vi "GetStringFromRing.vi"(7 "Index":bool, 8 "error in (no error)":errorcluster, 10 "Select Asset":i32, 11 "Ring in":refnum<vi>) -> (0 "error out":errorcluster, 3 "String":string)   [LabVIEW 2019]
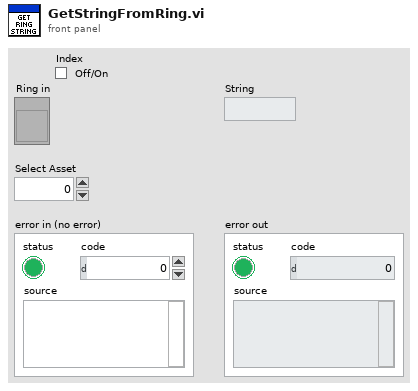
[diagram p1: front panel]
types:
  T1 = typedef "LVStringsAndValuesArrayTypeDef.ctl" = cluster{"String":string, "Value":ext}[]
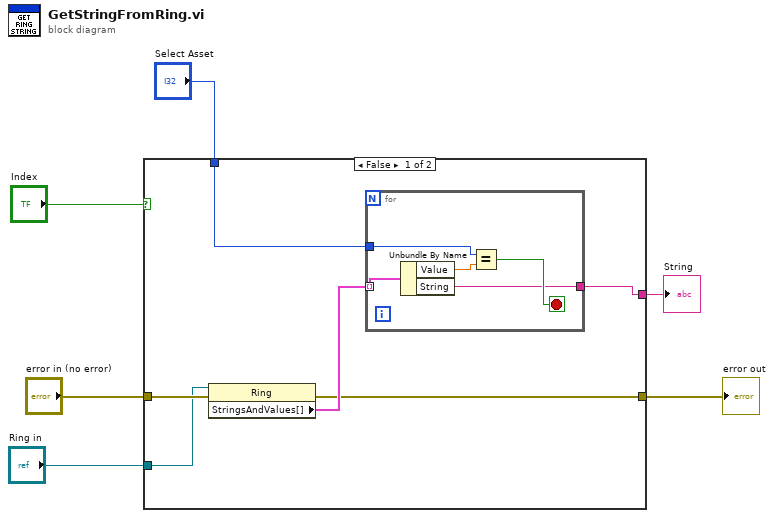
[diagram p0: block diagram]
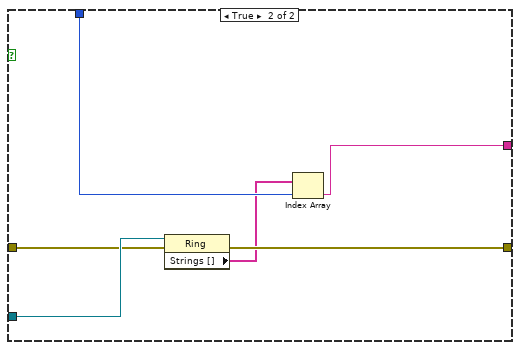
[diagram p2: hidden frame]
diagram:
  n1 = case shown="False" "Index" {
    tunnel: [w7 w23] -> w6
    tunnel: [w8 w22] -> w5
    tunnel: "Select Asset" -> [w9 w21]
    tunnel: "Ring in" -> [w11 w19]
    tunnel: "error in (no error)" -> [w12 w18]
    frame False {
      n2 = property class="Ring"(reference=w11, error in=w12) -> (error out=w7:errorcluster, "StringsAndValues[]"=w10:T1)  [unwired: 1 out]
      n3 = for {
        tunnel: w10 -> [w17] mode=indexing
        tunnel: w9 -> [w16]
        tunnel: [w13] -> w8
        stop <- w14 stop-if-true
        n4 = Unbundle By Name(w17) -> ("Value"=w15:ext, "String"=w13:string)
        n5 = Equal?(x=w16, y=w15) -> (x = y?=w14:bool)
      }
    }
    frame True {
      n6 = property class="Ring"(reference=w19, error in=w18) -> (error out=w23:errorcluster, "Strings []"=w20:string[])  [unwired: 1 out]
      n7 = Index Array(array=w20, index=w21) -> (element=w22:string)
    }
  }
  "error out" <- w6
  "String" <- w5
